vi "LVProjectShortcut_CreateNewWizard_GetWeight.vi"(11 "Wizard":T1) -> (3 "Weight":i32)   [LabVIEW 2017, in "LVProject Shortcut.lvlib"]
uses:
  <resource>/Framework/Providers/API/ItemRef.ctl
  LVProject Shortcut.lvlib
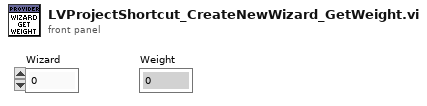
[diagram p1: front panel]
types:
  T1 = typedef "ItemRef.ctl" = u64
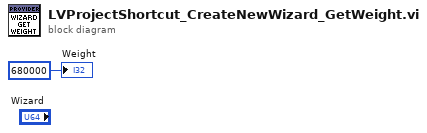
[diagram p0: block diagram]
diagram:
  "Weight" <- 680000 ("Weight")
